vi "HFRR ADV v01.vi"() -> ()   [LabVIEW 2025] (continued)
                  n3391 = local write "S 53"(w4387) -> ()
                }
                frame 53 {
                  n3392 = local write "S 54"(w4388) -> ()
                }
                frame 54 {
                  n3393 = local write "S 55"(w4389) -> ()
                }
                frame 55 {
                  n3394 = local write "S 56"(w4390) -> ()
                }
                frame 56 {
                  n3395 = local write "S 57"(w4391) -> ()
                }
                frame 57 {
                  n3396 = local write "S 58"(w4392) -> ()
                }
                frame 58 {
                  n3397 = local write "S 59"(w4393) -> ()
                }
                frame 59 {
                  n3398 = local write "S 60"(w4394) -> ()
                }
                frame 60 {
                  n3399 = local write "S 62"(w4395) -> ()
                }
                frame 61 {
                  n3400 = local write "S 63"(w4396) -> ()
                }
                frame 62 {
                  n3401 = local write "S 64"(w4397) -> ()
                }
                frame 63 {
                  n3402 = local write "S 65"(w4398) -> ()
                }
                frame 64 {
                  n3403 = local write "S 66"(w4399) -> ()
                }
                frame 65 {
                  n3404 = local write "S 67"(w4400) -> ()
                }
                frame 66 {
                  n3405 = local write "S 68"(w4401) -> ()
                }
                frame 67 {
                  n3406 = local write "S 69"(w4402) -> ()
                }
                frame 68 {
                  n3407 = local write "S 70"(w4403) -> ()
                }
                frame 69 {
                  n3408 = local write "S 71"(w4404) -> ()
                }
                frame 70 {
                  n3409 = local write "S 72"(w4405) -> ()
                }
                frame 71 {
                  n3410 = local write "S 73"(w4406) -> ()
                }
                frame 72 {
                  n3411 = local write "S 74"(w4407) -> ()
                }
                frame 73 {
                  n3412 = local write "S 75"(w4408) -> ()
                }
                frame 74 {
                  n3413 = local write "S 76"(w4409) -> ()
                }
                frame 75 {
                  n3414 = local write "S 77"(w4410) -> ()
                }
                frame 76 {
                  n3415 = local write "S 78"(w4411) -> ()
                }
                frame 77 {
                  n3416 = local write "S 79"(w4412) -> ()
                }
                frame 79 {
                  n3417 = property on="Sample Temperature ( °C )" class="XYGraph (strict)"("Y Scale.Name Label.Text"=w4413) -> ()  [unwired: 2 in, 2 out]
                }
                frame 80 {
                  n3418 = local write "S 81"(w4414) -> ()
                  n3419 = property on="Humidity ( %RH )" class="XYGraph (strict)"("Y Scale.Name Label.Text"=w4414) -> ()  [unwired: 2 in, 2 out]
                }
                frame 78 {
                  n3420 = property on="Air Temperature  ( °C )" class="XYGraph (strict)"("X Scale.Name Label.Text"=w4415) -> ()  [unwired: 2 in, 2 out]
                  n3421 = property on="Humidity ( %RH )" class="XYGraph (strict)"("X Scale.Name Label.Text"=w4415) -> ()  [unwired: 2 in, 2 out]
                  n3422 = property on="Sample Temperature ( °C )" class="XYGraph (strict)"("X Scale.Name Label.Text"=w4415) -> ()  [unwired: 2 in, 2 out]
                  n3423 = property on="Coefficient Of Friction" class="XYGraph (strict)"("X Scale.Name Label.Text"=w4415) -> ()  [unwired: 2 in, 2 out]
                }
                frame 81 {
                  n3424 = property on="Air Temperature  ( °C )" class="XYGraph (strict)"("Y Scale.Name Label.Text"=w4416) -> ()  [unwired: 2 in, 2 out]
                }
                frame 82 {
                  n3425 = local write "S 84"(w4417) -> ()
                }
                frame 83 {
                  n3426 = local write "S 85"(w4418) -> ()
                }
                frame 84 {
                  n3427 = local write "S 86"(w4419) -> ()
                }
                frame 85 {
                  n3428 = local write "S 87"(w4420) -> ()
                }
                frame 86 {
                  n3429 = local write "S 88"(w4421) -> ()
                }
                frame 87 {
                }
                frame 88 {
                  n3430 = local write "S 90"(w4423) -> ()
                }
                frame 89 {
                  n3431 = local write "S 91"(w4424) -> ()
                }
                frame 90 {
                  n3432 = local write "S 92"(w4425) -> ()
                }
                frame 91 {
                  n3433 = local write "S 93"(w4426) -> ()
                }
                frame 92 {
                  n3434 = local write "S 94"(w4427) -> ()
                }
                frame 93 {
                  n3435 = local write "S 95"(w4428) -> ()
                }
                frame 94 {
                  n3436 = local write "S 96"(w4429) -> ()
                }
                frame 95 {
                  n3437 = local write "S 97"(w4430) -> ()
                }
                frame 96 {
                  n3438 = local write "S 98"(w4431) -> ()
                }
                frame 97 {
                  n3439 = local write "S 99"(w4432) -> ()
                }
                frame 98 {
                  n3440 = local write "S 100"(w4433) -> ()
                }
                frame 99 {
                  n3441 = local write "S 101"(w4434) -> ()
                }
                frame 100 {
                  n3442 = local write "S 102"(w4435) -> ()
                }
                frame 101 {
                  n3443 = local write "S 103"(w4436) -> ()
                }
                frame 102 {
                  n3444 = local write "S 104"(w4437) -> ()
                }
                frame 103 {
                  n3445 = local write "S 105"(w4438) -> ()
                }
                frame 104 {
                  n3446 = local write "S 106"(w4439) -> ()
                }
                frame 105 {
                }
                frame 106 {
                  n3447 = property on="OK Button 17" class="Bool (strict)"("Boolean Text.Text"=w4440) -> ()  [unwired: 2 in, 2 out]
                }
                frame 107 {
                  n3448 = property on="OK Button 16" class="Bool (strict)"("Boolean Text.Text"=w4441) -> ()  [unwired: 2 in, 2 out]
                }
                frame 108 {
                  n3449 = property on="TITTLE" class="Str"("Caption.Text"=w4442) -> ()  [unwired: 2 in, 2 out]
                }
                frame 109 {
                  "String 30" <- w4443
                }
                frame 110 {
                  n3450 = property on="Test Date" class="Str"("Caption.Text"=w4444) -> ()  [unwired: 2 in, 2 out]
                  "String 31" <- w4444
                }
                frame 111 {
                  n3451 = property on="Sample ID" class="Str"("Caption.Text"=w4445) -> ()  [unwired: 2 in, 2 out]
                  "String 32" <- w4445
                }
                frame 112 {
                  n3452 = property on="Tested by" class="Str"("Caption.Text"=w4446) -> ()  [unwired: 2 in, 2 out]
                  "String 33" <- w4446
                }
                frame 113 {
                  n3453 = property on="System Configured Printers 2" class="Arr (strict)"("Caption.Text"=w4447) -> ()  [unwired: 2 in, 2 out]
                }
                frame 114 {
                  n3454 = property on="Selected Printer" class="Str"("Caption.Text"=w4448) -> ()  [unwired: 2 in, 2 out]
                }
                frame 115 {
                  n3455 = property on="Select Printer 3" class="DigNum (strict)"("Caption.Text"=w4449) -> ()  [unwired: 2 in, 2 out]
                }
                frame 116 {
                  n3456 = property on="Print" class="Bool (strict)"("Boolean Text.Text"=w4450) -> ()  [unwired: 2 in, 2 out]
                }
                frame 117 {
                  "String 41" <- w4451
                }
                frame 118 {
                  n3457 = property on="tested by" class="Str"("Caption.Text"=w4452) -> ()  [unwired: 2 in, 2 out]
                }
                frame 119 {
                }
                frame 120 {
                  n3458 = property on="Export" class="Bool (strict)"("Boolean Text.Text"=w4453) -> ()  [unwired: 2 in, 2 out]
                }
                frame 121 {
                }
                frame 122 {
                }
                frame 123 {
                  n3459 = property on="Select File Type" class="Enum (strict)"("Caption.Text"=w4456) -> ()  [unwired: 2 in, 2 out]
                }
                frame 124 {
                  n3460 = property on="s.NO" class="Str"("Caption.Text"=w4457) -> ()  [unwired: 2 in, 2 out]
                  "String 45" <- w4457
                }
                frame 125 {
                  n3461 = property on="trip1 8" class="Bool (strict)"("Boolean Text.Text"=w4458) -> ()  [unwired: 2 in, 2 out]
                }
                frame 126, Default {
                }
              }
            }
          }
          frame #1 {
            w4466 = TRUE ("Visible")
            n3462 = local read "S 91"() -> (w4483:string)
            n3463 = local read "S 90"() -> (w4482:string)
            n3464 = local read "S 88"() -> (w4481:string)
            n3465 = property on="File Path" class="Path"("Caption.Text"=w4482) -> ()  [unwired: 2 in, 2 out]
            n3466 = local read "S 71"() -> (w4476:string)
            n3467 = local read "S 86"() -> (w4478:string)
            n3468 = local read "S 85"() -> (w4479:string)
            n3469 = local read "S 87"() -> (w4477:string)
            n3470 = local read "S 84"() -> (w4480:string)
            n3471 = local read "S 103"() -> (w4465:string)
            n3472 = local read "S 104"() -> (w4464:string)
            n3473 = property on="Password" class="Str"("Caption.Text"=w4479) -> ()  [unwired: 2 in, 2 out]
            n3474 = property on="EDIT" class="Bool (strict)"("Boolean Text.Text"=w4476) -> ()  [unwired: 2 in, 2 out]
            n3475 = property on="SAVE" class="Bool (strict)"("Boolean Text.Text"=w4480) -> ()  [unwired: 2 in, 2 out]
            n3476 = Build Array(w4465, w4464) -> (w4463:string[])
            n3477 = property on="Heater Button" class="Bool (strict)"("Strings [4]"=w4463) -> ()  [unwired: 2 in, 2 out]
            n3478 = local read "S 92"() -> (w4475:string)
            n3479 = local read "S 93"() -> (w4474:string)
            n3480 = local read "S 105"() -> (w4461:string)
            n3481 = local read "S 106"() -> (w4460:string)
            n3482 = Build Array(w4475, w4474) -> ()  [unwired: 1 out]
            n3483 = Build Array(w4461, w4460) -> (w4462:string[])
            n3484 = local read "S 95"() -> (w4472:string)
            n3485 = local read "S 94"() -> (w4473:string)
            n3486 = local read "bs"() -> (w4488:string)
            n3487 = local read "as"() -> (w4489:string)
            n3488 = property on="Humidity" class="Bool (strict)"("Strings [4]"=w4462) -> ()  [unwired: 2 in, 2 out]
            n3489 = Concatenate Strings(w4488, "\r", w4489) -> ()  [unwired: 1 out]
            n3490 = property on="Rh After" class="DigNum (strict)"("Caption.Size to Text?"=TRUE ("Caption.Size to Text")) -> ()  [unwired: 2 in, 2 out]
            n3491 = local read "S 48"() -> (w4512:string)
            n3492 = local read "S 50"() -> (w4510:string)
            n3493 = local read "S 51"() -> (w4509:string)
            n3494 = local read "S 49"() -> (w4511:string)
            n3495 = local read "S 52"() -> (w4508:string)
            n3496 = local read "as"() -> (w4493:string)
            n3497 = local read "bs"() -> (w4494:string)
            n3498 = local read "S 56"() -> (w4507:string)
            n3499 = local read "S 57"() -> (w4506:string)
            n3500 = local read "S 58"() -> (w4505:string)
            n3501 = local read "S 59"() -> (w4504:string)
            n3502 = property on="OPEN" class="Bool (strict)"("Boolean Text.Text"=w4508) -> ()  [unwired: 2 in, 2 out]
            n3503 = property on="OPEN 1" class="Bool (strict)"("Boolean Text.Text"=w4512) -> ()  [unwired: 2 in, 2 out]
            n3504 = property on="OPEN 2" class="Bool (strict)"("Boolean Text.Text"=w4511) -> ()  [unwired: 2 in, 2 out]
            n3505 = property on="OPEN 3" class="Bool (strict)"("Boolean Text.Text"=w4510) -> ()  [unwired: 2 in, 2 out]
            n3506 = property on="OPEN 4" class="Bool (strict)"("Boolean Text.Text"=w4509) -> ()  [unwired: 2 in, 2 out]
            n3507 = Concatenate Strings(w4494, "\r", w4493) -> ()  [unwired: 1 out]
            n3508 = local read "S 102"() -> (w4467:string)
            n3509 = property on="КОФ1" class="DigNum (strict)"("Caption.Text"=w4507) -> ()  [unwired: 2 in, 2 out]
            n3510 = local read "S 98"() -> (w4471:string)
            n3511 = local read "S 99"() -> (w4470:string)
            n3512 = local read "S 100"() -> (w4469:string)
            n3513 = local read "S 101"() -> (w4468:string)
            n3514 = property on="КОФ2" class="DigNum (strict)"("Caption.Text"=w4506) -> ()  [unwired: 2 in, 2 out]
            n3515 = property on="КОФ3" class="DigNum (strict)"("Caption.Text"=w4505) -> ()  [unwired: 2 in, 2 out]
            n3516 = property on="КОФ4" class="DigNum (strict)"("Caption.Text"=w4504) -> ()  [unwired: 2 in, 2 out]
            n3517 = local read "bs"() -> (w4492:string)
            n3518 = local read "as"() -> (w4491:string)
            n3519 = local read "S 60"() -> (w4503:string)
            n3520 = local read "S 54"() -> (w4513:string)
            n3521 = Concatenate Strings(w4492, "\r", w4491) -> ()  [unwired: 1 out]
            n3522 = Concatenate Strings(w4513, w4503) -> ()  [unwired: 1 out]
            n3523 = local read "S 77"() -> (→"String 43":string)
            n3524 = local read "S 76"() -> (w4486:string)
            n3525 = local read "S 78"() -> (w4485:string)
            n3526 = local read "S 71"() -> (w4497:string)
            n3527 = local read "S 66"() -> (w4502:string)
            n3528 = local read "S 67"() -> (w4501:string)
            n3529 = local read "S 68"() -> (w4500:string)
            n3530 = local read "S 69"() -> (w4499:string)
            n3531 = local read "S 70"() -> (w4498:string)
            n3532 = property on="AIR TEMP" class="DigNum (strict)"("Caption.Text"=w4485) -> ()  [unwired: 2 in, 2 out]
            n3533 = property on="Set Strk" class="DigNum (strict)"("Caption.Text"=w4486) -> ()  [unwired: 2 in, 2 out]
            n3534 = property on="SPEED OUT:" class="DigNum (strict)"("Caption.Text"=w4500) -> ()  [unwired: 2 in, 2 out]
            n3535 = property on="EDIT" class="Bool (strict)"("Boolean Text.Text"=w4497) -> ()  [unwired: 2 in, 2 out]
            n3536 = local read "S 79"() -> (w4484:string)
          }
          frame #2 {
          }
        }
        n3537 = local write "Lan flag"(10.0 ("Lan flag")) -> ()
      }
      frame Enabled {
      }
    }
    n3538 = Wait (ms)(milliseconds to wait=u32 2000) -> ()  [unwired: 1 out]
    n3539 = local read "Quit"() -> (w4287:bool)
  }
  n3540 = while {
    shift-right: [w4519] -> _
    shift-left: _ -> [w4520]
    shift-right: [w4517] -> _
    shift-left: T18 {"Read Heave and Surge"="", "Bytes at Heave Port"=0.0, "Heave and Surge COM Port:"="COM9", "Com Port 2"="COM7", "Residual Due"="", "Heave COM Status 2"=TRUE, "Heave COM Status"=TRUE, "Port 2"=TRUE, "Sway PPR"=6400.0, "Surge PPR"=6400.0, "Heave PPR"=6400.0, "Sway Pitch"=2.0, "Surge Pitch"=3.0, "Heave Pitch"=4.0, "Sway Pulses/mm"=320.0, "Surge Pulses/mm"=1600.0, "Heave Pulses/mm"=1600.0, "inner loop"=0.0, "Read Heave and Surge 2"="", "String 36"="", "Write S"=FALSE, "WriteCC1"=[""], "Heave COM Loop"=0, "LastCom"="", "EXIT"=FALSE, "Error Heave"={"status"=TRUE, "code"=-1073807343, "source"=""}} -> [w4516]
    shift-right: [w4514] -> _
    shift-left: enum16{"init", "MAIN", "Panel Close"}."init" -> [w4515]
    stop <- w4518 stop-if-true
    # "HUMIDITY LOOP LOGIC"
    n3541 = case shown="\"MAIN\"" w4515 {
      tunnel: w4520 -> [w4534 w4558 w4622 w4624]
      tunnel: [w4529 w4545 w4622 w4624] -> w4519
      tunnel: [_ _ TRUE _] -> w4518
      tunnel: [w4526 w4543 w4620 w4623] -> w4517
      tunnel: w4516 -> [w4531 w4557 w4620 w4623]
      tunnel: [enum16{"init", "MAIN", "Panel Close"}."MAIN" w4552 _ _] -> w4514
      frame "init" {
        n3542 = local read "C3 :"() -> (w4521:refnum<visa-resource-name>)
        n3543 = Bundle By Name(cluster=w4531, "Heave and Surge COM Port:"=w4521) -> (w4530:T18)
        n3544 = call "Instrument fgv uno.vi"("Enum"=T31."INIT", "error in (no error) 2"=w4534, "INPUT"=w4530) -> ("error"=w4532:errorcluster, "output"=w4528:T18)  [unwired: 6 in, 1 out]
        n3545 = case shown="Error" w4532 {
          selector: w4532 -> [w4536 _]
          tunnel: [w4536 w4540] -> w4529
          tunnel: w4528 -> [w4535 w4538]
          tunnel: [w4535 w4537] -> w4527
          frame No Error {
          }
          frame Error {
            n3546 = call "Instrument fgv uno.vi"("Enum"=T31."ERROR INIT", "INPUT"=w4538) -> ("error"=w4541:errorcluster, "output"=w4537:T18)  [unwired: 7 in, 1 out]
            n3547 = call <vilib>:"Clear Errors.vi"("error in (no error)"=w4541) -> ("error out"=w4540:errorcluster)  [unwired: 5 in, 1 out]
          }
        }
        n3548 = local read "LastCom Humidity"() -> (w4524:string)
        n3549 = Unbundle By Name(w4527) -> ("Heave COM Status 2"=→"COM Status":bool, "Error Heave"=→"Error":errorcluster)  [unwired: 1 out]
        n3550 = Bundle By Name(cluster=w4527, "LastCom"=w4524) -> (w4526:T18)
      }
      frame "MAIN" {
        n3551 = Unbundle By Name(w4557) -> ("Com Port 2"=w4547:refnum<visa-resource-name>)
        n3552 = local read "C3 :"() -> (w4548:refnum<visa-resource-name>)
        n3553 = local write "COM Port Humidity :"(w4547) -> ()
        n3554 = Bundle By Name(cluster=w4557, "Heave and Surge COM Port:"=w4548) -> (w4556:T18)
        n3555 = Equal?(x=w4547, y=w4548) -> (x = y?=w4561:bool)
        n3556 = case shown="True" w4561 {
          tunnel: [w4576 w4593] -> w4546
          tunnel: w4558 -> [w4577 w4599]
          tunnel: w4556 -> [w4575 w4597]
          tunnel: [w4574 w4592] -> w4544
          frame False {
            n3557 = call <vilib>:"Clear Errors.vi"("error in (no error)"=w4577) -> ("error out"=w4573:errorcluster)  [unwired: 5 in, 1 out]
            n3558 = call "Instrument fgv uno.vi"("Enum"=T31."ERROR INIT", "error in (no error) 2"=w4573, "INPUT"=w4575) -> ("error"=w4579:errorcluster, "output"=w4574:T18)  [unwired: 6 in, 1 out]
            n3559 = call <vilib>:"Clear Errors.vi"("error in (no error)"=w4579) -> ("error out"=w4576:errorcluster)  [unwired: 5 in, 1 out]
          }
          frame True {
            n3560 = call "Instrument fgv uno.vi"("Enum"=T31."READ", "error in (no error) 2"=w4599, "INPUT"=w4597) -> ("error"=w4598:errorcluster, "output"=w4591:T18)  [unwired: 6 in, 1 out]
            n3561 = Bundle By Name(cluster=w4591, "String 36"="WRITE HUMIDITY") -> (w4590:T18)
            n3562 = case shown="True" "Write Humidity" {
              selector: "Write Humidity" -> [_ w4619]
              tunnel: w4598 -> [w4612 w4618]
              tunnel: [w4612 w4617] -> w4588
              tunnel: w4590 -> [w4611 w4615]
              tunnel: [w4611 w4614] -> w4587
              frame False {
              }
              frame True {
                n3563 = Not(x=w4619) -> (.not. x?=w4613:bool)
                n3564 = local write "Write Humidity"(w4613) -> ()
                n3565 = call "Instrument fgv uno.vi"("Enum"=T31."MANUAL WRITE", "error in (no error) 2"=w4618, "INPUT"=w4615) -> ("error"=w4617:errorcluster, "output"=w4614:T18)  [unwired: 6 in, 1 out]
              }
            }
            n3566 = Array Size(array="WriteHumidity") -> (size(s)=w4585:i32)
            n3567 = Greater Than 0?(x=w4585) -> (x > 0?=w4584:bool)
            n3568 = call "Instrument fgv uno.vi"("Enum"=T31."WRITE", "error in (no error) 2"=w4588, "WriteCC1"="WriteHumidity", "INPUT"=w4587) -> ("error"=w4595:errorcluster, "WriteCC1 2"=w4586:string[], "output"=w4594:T18)  [unwired: 5 in]
            n3569 = case shown="True" w4584 {
              tunnel: w4586 -> [_ w4601]
              frame False {
              }
              frame True {
                n3570 = local write "WriteHumidity"(w4601) -> ()
              }
            }
            n3571 = case shown="No Error" w4595 {
              selector: w4595 -> [w4602 w4605]
              tunnel: w4594 -> [w4603 w4610]
              tunnel: [w4603 w4609] -> w4592
              tunnel: [w4602 w4607] -> w4593
              frame No Error {
              }
              frame Error {
                n3572 = call <vilib>:"Clear Errors.vi"("error in (no error)"=w4605) -> ("error out"=w4604:errorcluster)  [unwired: 5 in, 1 out]
                n3573 = call "Instrument fgv uno.vi"("Enum"=T31."ERROR INIT", "error in (no error) 2"=w4604, "INPUT"=w4610) -> ("error"=w4608:errorcluster, "output"=w4609:T18)  [unwired: 6 in, 1 out]
                n3574 = call <vilib>:"Clear Errors.vi"("error in (no error)"=w4608) -> ("error out"=w4607:errorcluster)  [unwired: 5 in, 1 out]
              }
            }
            n3575 = Unbundle By Name(w4592) -> ("LastCom"=→"LastCom Humidity":string, "Read Heave and Surge"=→"Read HUMIDITY":string)
          }
        }
        n3576 = Unbundle By Name(w4544) -> ("Heave COM Status 2"=w4560:bool, "Error Heave"=w4549:errorcluster, "Bytes at Heave Port"=→"Bytes at Humidity Port  2":dbl)  [unwired: 1 out]
        n3577 = Unbundle By Name(w4549) -> ("status"=→"Humidity Port":bool)
        n3578 = Not(x=w4560) -> (.not. x?=w4550:bool)
        n3579 = local write "Error"(w4549) -> ()
        n3580 = local read "Quit"() -> (w4553:bool)
        n3581 = local write "COM Status"(w4550) -> ()
        n3582 = Select(t=enum16{"init", "MAIN", "Panel Close"}."Panel Close", s=w4553, f=enum16{"init", "MAIN", "Panel Close"}."MAIN") -> (s? t:f=w4552:enum16{"init", "MAIN", "Panel Close"})
        n3583 = local read "Humidity 2"() -> (w4542:bool)
        n3584 = case shown="True" w4542 {
          selector: w4542 -> [_ w4564]
          tunnel: w4546 -> [w4562 w4569]
          tunnel: [w4562 w4568] -> w4545
          tunnel: w4544 -> [w4563 w4567]
          tunnel: [w4563 w4566] -> w4543
          frame False {
          }
          frame True {
            n3585 = Not(x=w4564) -> (.not. x?=→"Humidity 2":bool)
            n3586 = call <vilib>:"Clear Errors.vi"("error in (no error)"=w4569) -> ("error out"=w4572:errorcluster)  [unwired: 5 in, 1 out]
            n3587 = call "Instrument fgv uno.vi"("Enum"=T31."ERROR INIT", "error in (no error) 2"=w4572, "INPUT"=w4567) -> ("error"=w4570:errorcluster, "output"=w4566:T18)  [unwired: 6 in, 1 out]
            n3588 = call <vilib>:"Clear Errors.vi"("error in (no error)"=w4570) -> ("error out"=w4568:errorcluster)  [unwired: 5 in, 1 out]
          }
        }
      }
      frame "Panel Close" {
      }
      frame Default {
      }
    }
  }
  n3589 = while {
    stop <- w4626 stop-if-true
    n3590 = call <vilib>:"High Resolution Polling Wait.vi"("seconds to wait"=0.05) -> ()  [unwired: 10 in, 1 out]
    n3591 = disable-structure shown="Enabled" {
      frame Disabled {
        n3592 = local read "Read HUMIDITY"() -> (w4627:string)
        n3593 = Spreadsheet String To Array(delimiter (Tab)=",", format string="", spreadsheet string=w4627, array type (2D Dbl)=string[] []) -> (array=w4646:string[])
        n3594 = for {
          tunnel: w4646 -> [w4655] mode=indexing
          tunnel: string[] ["STATE;", "SET;", "RH;", "T;", "AMB_RH;", "AMB_T;", "PUMP;", "FAN_IN;", "FAN_OUT;", "DEHUM;", "CURRENT;", "STALL;"] -> [w4654] mode=indexing
          tunnel: [w4653] -> w4645 mode=indexing
          n3595 = Match Pattern(string=w4655, regular expression=w4654) -> (after substring=w4653:string)  [unwired: 1 in, 3 out]
        }
        n3596 = Index Array(array=w4645) -> (element #1=w4644:string, element #2=w4643:string, element #3=w4635:string, element #4=w4634:string, element #5=w4633:string, element #6=w4642:string, element #7=w4641:string, element #8=w4640:string, element #9=w4639:string, element #10=w4638:string, element #11=w4637:string, element #12=w4636:string)  [unwired: 12 in]
        n3597 = Fract/Exp String To Number(string=w4635) -> (number=w4628:dbl)  [unwired: 3 in, 1 out]
        n3598 = Fract/Exp String To Number(string=w4633) -> (number=w4632:dbl)  [unwired: 3 in, 1 out]
        n3599 = local write "Ambient Humidity :"(w4632) -> ()
        n3600 = Equal?(x=w4628, y=0.0) -> (x = y?=w4630:bool)
        n3601 = case shown="True" w4630 {
          tunnel: [w4651 w4652] -> w4629
          tunnel: w4628 -> [w4651 _]
          frame False {
            (unwired) 0.0
            "Humidity temp" <- w4651
          }
          frame True {
            n3602 = local read "Humidity temp"() -> (w4652:dbl)
          }
        }
        "RH Numeric:" <- w4629
      }
      frame Enabled {
        n3603 = local read "Read HUMIDITY"() -> (w4675:string)
        n3604 = Spreadsheet String To Array(delimiter (Tab)=",", format string="", spreadsheet string=w4675, array type (2D Dbl)=dbl[] []) -> (array=w4671:dbl[])
        n3605 = Index Array(array=w4671) -> (element #1=→"STATE :":dbl, element #2=→"SET :":dbl, element #3=w4656:dbl, element #4=→"T :":dbl, element #5=→"AMB_RH :":dbl, element #6=→"AMB_T :":dbl, element #7=→"PUMP :":dbl, element #8=→"FAN_IN :":dbl, element #9=→"FAN_OUT :":dbl, element #10=→"DEHUM :":dbl, element #11=→"CURRENT :":dbl, element #12=→"STALL":dbl)  [unwired: 12 in]
        "RH :" <- w4656
        n3606 = Equal?(x=w4656, y=0.0) -> (x = y?=w4659:bool)
        n3607 = case shown="False" w4659 {
          tunnel: [w4676 w4677] -> w4660
          tunnel: w4656 -> [w4676 _]
          frame False {
            "Humidity temp 2" <- w4676
          }
          frame True {
            n3608 = local read "Humidity temp 2"() -> (w4677:dbl)
          }
        }
        n3609 = local write "RH Numeric:"(w4660) -> ()
      }
    }
    n3610 = local read "Quit"() -> (w4626:bool)
  }
  n3611 = while {
    shift-right: [w4683] -> _
    shift-left: _ -> [w4684]
    shift-right: [w4681] -> _
    shift-left: T20 {"Read Uno"="", "Bytes at Heave Port"=0.0, "UNO COM Port:"="COM9", "UNO COM Port: 2"="COM7", "Residual Due"="", "UNO COM Status 2"=TRUE, "UNO COM Status"=TRUE, "Port 2"=TRUE, "Sway PPR"=6400.0, "Surge PPR"=6400.0, "Heave PPR"=6400.0, "Sway Pitch"=2.0, "Surge Pitch"=3.0, "Heave Pitch"=4.0, "Sway Pulses/mm"=320.0, "Surge Pulses/mm"=1600.0, "Heave Pulses/mm"=1600.0, "inner loop"=0.0, "Read Heave and Surge 2"="", "String 36"="", "Write S"=FALSE, "WriteCC1"=[""], "Heave COM Loop"=0, "LastCom"="", "EXIT"=FALSE, "Error Heave"={"status"=TRUE, "code"=-1073807343, "source"=""}} -> [w4680]
    shift-right: [w4678] -> _
    shift-left: enum16{"init", "MAIN", "Panel Close"}."init" -> [w4679]
    stop <- w4682 stop-if-true
    # "UNO CODE LOGIC"
    n3612 = case shown="\"MAIN\"" w4679 {
      tunnel: w4684 -> [w4698 w4717 w4773 w4775]
      tunnel: [w4693 w4722 w4773 w4775] -> w4683
      tunnel: [_ _ TRUE _] -> w4682
      tunnel: [w4689 w4720 w4771 w4774] -> w4681
      tunnel: w4680 -> [w4695 w4716 w4771 w4774]
      tunnel: [enum16{"init", "MAIN", "Panel Close"}."MAIN" w4711 _ _] -> w4678
      frame "init" {
        n3613 = local read "Com Port 1"() -> (w4685:refnum<visa-resource-name>)
        n3614 = Bundle By Name(cluster=w4695, "UNO COM Port:"=w4685) -> (w4694:T20)
        n3615 = call "Instrument fgv.vi"("Enum"=T31."INIT", "error in (no error) 2"=w4698, "INPUT"=w4694) -> ("error"=w4696:errorcluster, "output"=w4692:T18)  [unwired: 6 in, 1 out]
        n3616 = case shown="Error" w4696 {
          selector: w4696 -> [w4700 _]
          tunnel: [w4700 w4704] -> w4693
          tunnel: w4692 -> [w4699 w4702]
          tunnel: [w4699 w4701] -> w4690
          frame No Error {
          }
          frame Error {
            n3617 = call "Instrument fgv.vi"("Enum"=T31."ERROR INIT", "INPUT"=w4702) -> ("error"=w4705:errorcluster, "output"=w4701:T18)  [unwired: 7 in, 1 out]
            n3618 = call <vilib>:"Clear Errors.vi"("error in (no error)"=w4705) -> ("error out"=w4704:errorcluster)  [unwired: 5 in, 1 out]
          }
        }
        n3619 = local read "LastCom UNO"() -> (w4687:string)
        n3620 = Unbundle By Name(w4690) -> ("Heave COM Status 2"=→"Instrument Status":bool, "Error Heave"=→"Error  2":errorcluster)  [unwired: 1 out]
        n3621 = Bundle By Name(cluster=w4690, "LastCom"=w4687) -> (w4689:T18)
      }
      frame "MAIN" {
        n3622 = Unbundle By Name(w4716) -> ("UNO COM Port: 2"=w4706:refnum<visa-resource-name>)
        n3623 = local read "Com Port 1"() -> (w4707:refnum<visa-resource-name>)
        n3624 = local write "COM Port UNO :"(w4706) -> ()
        n3625 = Equal?(x=w4706, y=w4707) -> (x = y?=w4723:bool)
        n3626 = Bundle By Name(cluster=w4716, "UNO COM Port:"=w4707) -> (w4715:T20)
        n3627 = case shown="True" w4723 {
          tunnel: [w4727 w4744] -> w4722
          tunnel: w4717 -> [w4728 w4750]
          tunnel: w4715 -> [w4726 w4748]
          tunnel: [w4725 w4743] -> w4720
          frame False {
            n3628 = call <vilib>:"Clear Errors.vi"("error in (no error)"=w4728) -> ("error out"=w4724:errorcluster)  [unwired: 5 in, 1 out]
            n3629 = call "Instrument fgv.vi"("Enum"=T31."ERROR INIT", "error in (no error) 2"=w4724, "INPUT"=w4726) -> ("error"=w4730:errorcluster, "output"=w4725:T18)  [unwired: 6 in, 1 out]
            n3630 = call <vilib>:"Clear Errors.vi"("error in (no error)"=w4730) -> ("error out"=w4727:errorcluster)  [unwired: 5 in, 1 out]
          }
          frame True {
            n3631 = call "Instrument fgv.vi"("Enum"=T31."READ", "error in (no error) 2"=w4750, "INPUT"=w4748) -> ("error"=w4749:errorcluster, "output"=w4742:T18)  [unwired: 6 in, 1 out]
            n3632 = Bundle By Name(cluster=w4742, "String 36"="WRITE UNO") -> (w4741:T18)
            n3633 = case shown="True" "Write" {
              selector: "Write" -> [_ w4765]
              tunnel: w4749 -> [w4763 w4770]
              tunnel: [w4763 w4769] -> w4739
              tunnel: w4741 -> [w4762 w4767]
              tunnel: [w4762 w4766] -> w4738
              frame False {
              }
              frame True {
                n3634 = Not(x=w4765) -> (.not. x?=w4764:bool)
                n3635 = local write "Write"(w4764) -> ()
                n3636 = call "Instrument fgv.vi"("Enum"=T31."MANUAL WRITE", "error in (no error) 2"=w4770, "INPUT"=w4767) -> ("error"=w4769:errorcluster, "output"=w4766:T18)  [unwired: 6 in, 1 out]
              }
            }
            n3637 = Array Size(array="Write UNO") -> (size(s)=w4736:i32)
            n3638 = Greater Than 0?(x=w4736) -> (x > 0?=w4735:bool)
            n3639 = call "Instrument fgv.vi"("Enum"=T31."WRITE", "error in (no error) 2"=w4739, "WriteCC1"="Write UNO", "INPUT"=w4738) -> ("error"=w4746:errorcluster, "WriteCC1 2"=w4737:string[], "output"=w4745:T18)  [unwired: 5 in]
            n3640 = case shown="True" w4735 {
              tunnel: w4737 -> [_ w4752]
              frame False {
              }
              frame True {
                n3641 = local write "Write UNO"(w4752) -> ()
              }
            }
            n3642 = case shown="Error" w4746 {
              selector: w4746 -> [w4753 w4756]
              tunnel: w4745 -> [w4754 w4761]
              tunnel: [w4754 w4760] -> w4743
              tunnel: [w4753 w4758] -> w4744
              frame No Error {
              }
              frame Error {
                n3643 = call <vilib>:"Clear Errors.vi"("error in (no error)"=w4756) -> ("error out"=w4755:errorcluster)  [unwired: 5 in, 1 out]
                n3644 = call "Instrument fgv.vi"("Enum"=T31."ERROR INIT", "error in (no error) 2"=w4755, "INPUT"=w4761) -> ("error"=w4759:errorcluster, "output"=w4760:T18)  [unwired: 6 in, 1 out]
                n3645 = call <vilib>:"Clear Errors.vi"("error in (no error)"=w4759) -> ("error out"=w4758:errorcluster)  [unwired: 5 in, 1 out]
              }
            }
            n3646 = Unbundle By Name(w4743) -> ("LastCom"=→"LastCom UNO":string, "Read Heave and Surge"=→"Read UNO":string)
          }
        }
        n3647 = Unbundle By Name(w4720) -> ("Heave COM Status 2"=w4721:bool, "Heave COM Status"=w4710:bool, "Error Heave"=w4708:errorcluster, "Bytes at Heave Port"=→"Bytes at Humidity Port":dbl)
        n3648 = Not(x=w4710) -> (.not. x?=w4718:bool)
        n3649 = Not(x=w4721) -> (.not. x?=w4709:bool)
        n3650 = local write "Instrument Status"(w4718) -> ()
        n3651 = local write "Error  2"(w4708) -> ()
        n3652 = local write "Port 1a"(w4710) -> ()
        n3653 = local read "Quit"() -> (w4712:bool)
        n3654 = local write "COM Status"(w4709) -> ()
        n3655 = Select(t=enum16{"init", "MAIN", "Panel Close"}."Panel Close", s=w4712, f=enum16{"init", "MAIN", "Panel Close"}."MAIN") -> (s? t:f=w4711:enum16{"init", "MAIN", "Panel Close"})
      }
      frame "Panel Close" {
      }
      frame Default {
      }
    }
  }
